vi "LANC.vi"() -> ()   [LabVIEW 2020]
panel:
  in  "Tab.Main":enum32{"Controls", "Debugging"}(tab)
  in  "Rx.Status.Byte1":u8(ring) caption="Status" items=[""=0, "No Tape"=1, "Fast Forwarding"=3, "Rewinding"=131, "Stopped - Tape Beginning"=114, "Stopped"=2, "Recording"=4, "Playing"=6]
  in  "Rx.Status.Byte0":u8(ring) caption="Status" items=[""=0, "No Tape"=1, "Fast Forwarding"=3, "Rewinding"=131, "Stopped - Tape Beginning"=114, "Stopped"=2, "Recording"=4, "Playing"=6]
  in  "Power.Off":bool
  in  "Power.On":bool caption="Power On"
  in  "Zoom.Out":bool
  in  "Zoom.Speed":u8(knob) scale=0.0..7.0
  in  "Zoom.In":bool
  in  "Record.Stop":bool
  in  "Record.Start":bool caption="Record: Start"
  in  "Repetition.Period":u32 max=0
  in  "ControlName.Add":bool
  in  "ControlName.New":string caption="Control Name: New"
  in  "Command.Save":bool
  in  "Control.Names":u16(ring) caption="Control Names" items=["Power.On", "Power.Off", "Record.Start", "Record.Stop", "Zoom.In_0", "Zoom.In_1", "Zoom.In_2", "Zoom.In_3", "Zoom.In_4", "Zoom.In_5", "Zoom.In_6", "Zoom.In_7", "Zoom.Out_0", "Zoom.Out_1", "Zoom.Out_2", "Zoom.Out_3", "Zoom.Out_4", "Zoom.Out_5", "Zoom.Out_6", "Zoom.Out_7"]
  in  "COM Port":refnum<visa-resource-name>="COM3"
  out "LANC.Rx":string[](array[string])
  in  "LANC.Rx.DisplayType":bool caption="Display Type"
  in  "Clear":bool
  in  "Update":bool=TRUE
  in  "Interrapt":bool
  in  "Command.ASCII.Send":bool
  in  "Command.ASCII":string caption="Command (ASCII)"
  in  "Big/LittleEndian":bool
  out "Binary Array.NumericVal":u8 caption="Numeric" format="%02x"
  in  "Binary Array":bool[](array[boolean])=[FALSE, FALSE, FALSE, TRUE, FALSE, TRUE, FALSE, FALSE]
  out "error out":errorcluster
  in  "Exit":bool
  # "Controls"
  # "Tx"
  # "Rx"
  # "="
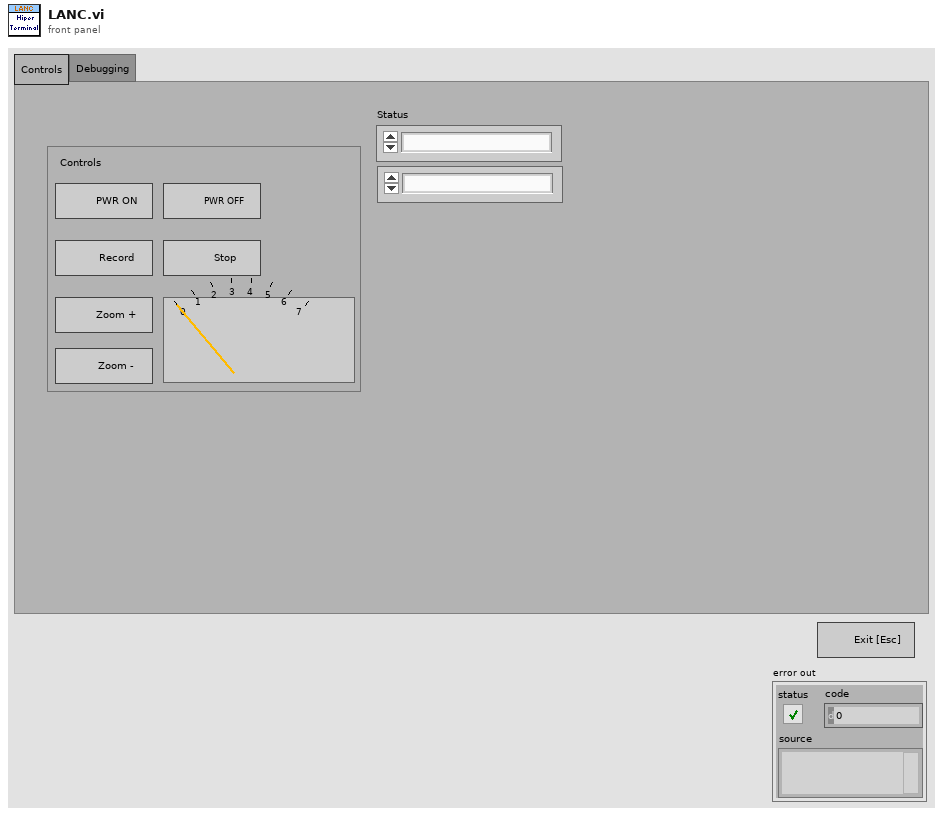
[diagram p1: front panel]
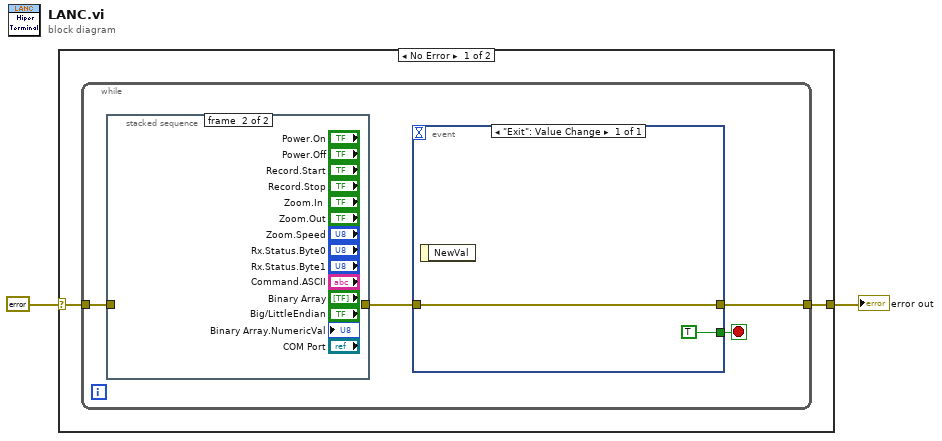
[diagram p0: block diagram]
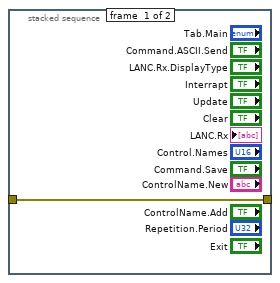
[diagram p2: hidden frame]
diagram:
  n1 = case shown="No Error" errorcluster {"status"=FALSE, "code"=0, "source"=""} ("error in (no error)") {
    selector: errorcluster {"status"=FALSE, "code"=0, "source"=""} ("error in (no error)") -> [w4 w12]
    tunnel: [w3 w12] -> w2
    frame No Error {
      n2 = while {
        tunnel: w4 -> [w8]
        tunnel: [w6] -> w3
        stop <- w5 stop-if-true
        n3 = stacked-sequence {
          tunnel: [w11 _] -> w7
          tunnel: w8 -> [w11 _]
          frame #0 {
          }
          frame #1 {
          }
        }
        n4 = event shown="[0] \"Exit\": Value Change" {
          selector: _ -> [_]
          dyn-events: _ -> [_]
          timeout: _ -> [_]
          tunnel: w7 -> [w10]
          tunnel: [w10] -> w6
          tunnel: [TRUE] -> w5
          event "Exit": Value Change {
            n5 = event-data() -> ()  [unwired: 1 in, 1 out]
          }
        }
      }
    }
    frame Error {
    }
  }
  "error out" <- w2
